vi "Inverse f Filter.vi"   [LabVIEW 2014, in "NI_AALBase.lvlib"]
doc: "Designs and implements an IIR filter whose magnitude-squared response is inversely proportional to frequency over a specified frequency range. This inverse-f filter is typically used to colorize spectrally flat, or white, noise. Wire data to the <B>X</B> input to determine the polymorphic instance to use or manually select the instance."
uses:
  NI_AALBase.lvlib
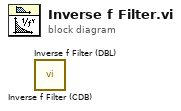
[diagram p0: block diagram]
diagram:
  n1 = call "Inverse f Filter (CDB).vi"() -> ()  [unwired: 7 in, 5 out]
  n2 = call "Inverse f Filter (DBL).vi"() -> ()  [unwired: 7 in, 5 out]
